vi "Binary Operation.vi"(4 "Function":u8(ring) items=["plus_saturated", "minus_saturated", "multiplies", "divides", "modulus", "equal_to", "not_equal_to", "greater", "greater_equal", "less", "less_equal", "logical_and", "logical_or", "bitwise_and", "bitwise_or"], 5 "Error":string, 6 "Output Image":T1={"Image ID"=0, "Channel ID"=-1}, 7 "Input Image 2":T1={"Image ID"=0, "Channel ID"=-1}, 8 "Input Image 1":T1={"Image ID"=0, "Channel ID"=-1}) -> (0 "Error":string, 1 "Output Image":T1={"Image ID"=0, "Channel ID"=-1}, 2 "Input Image 2":T1={"Image ID"=0, "Channel ID"=-1}, 3 "Input Image 1":T1={"Image ID"=0, "Channel ID"=-1})   [LabVIEW 2011, in "labvvis.lvlib"]
uses:
  <userlib>/labvvis/labvvis.lvlib
  <userlib>/labvvis/VVIS Image.ctl
  labvvis.framework
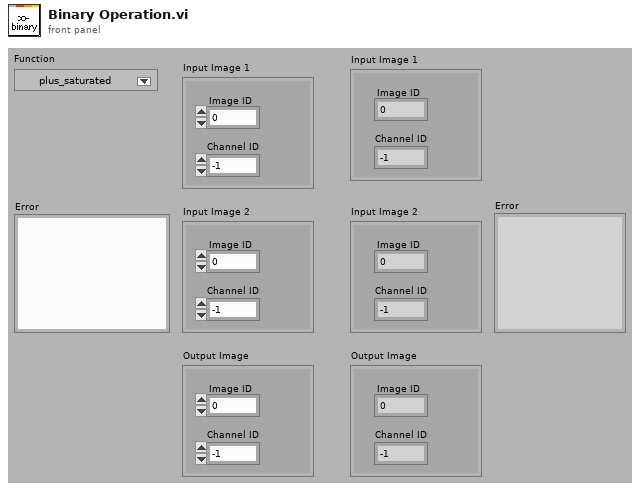
[diagram p1: front panel]
types:
  T1 = typedef "labvvis.lvlib/VVIS Image.ctl" = cluster{"Image ID":i16, "Channel ID":i16}
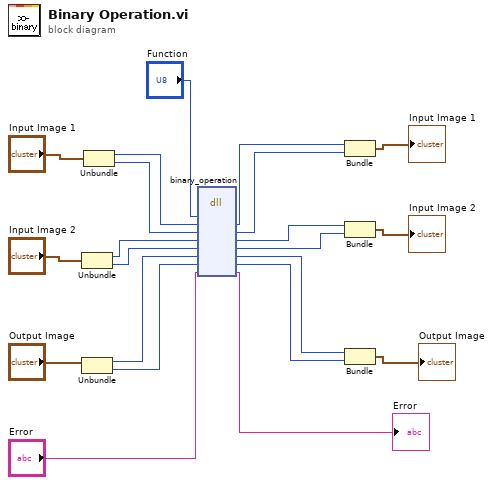
[diagram p0: block diagram]
diagram:
  n1 = Unbundle("Input Image 2") -> ("Image ID"=w15:i16, "Channel ID"=w14:i16)
  n2 = Unbundle("Output Image") -> ("Image ID"=w13:i16, "Channel ID"=w12:i16)
  n3 = Unbundle("Input Image 1") -> ("Image ID"=w17:i16, "Channel ID"=w16:i16)
  n4 = dll-call lib="labvvis.framework" fn="binary_operation"("function"="Function", "src1"=w17, "cid1"=w16, "src2"=w15, "cid2"=w14, "out"=w13, "ocid"=w12, "error"="Error") -> ("src1"=w10:i16, "cid1"=w9:i16, "src2"=w8:i16, "cid2"=w7:i16, "out"=w6:i16, "ocid"=w5:i16, "error"=→"Error":string)  [unwired: 5 in, 2 out]
  n5 = Bundle("src1"=w10, "cid1"=w9) -> (→"Input Image 1":cluster{"src1":i16, "cid1":i16})  [unwired: 1 in]
  n6 = Bundle("src2"=w8, "cid2"=w7) -> (→"Input Image 2":cluster{"src2":i16, "cid2":i16})  [unwired: 1 in]
  n7 = Bundle("out"=w6, "ocid"=w5) -> (→"Output Image":cluster{"out":i16, "ocid":i16})  [unwired: 1 in]
